vi "Collector Lift.vi"(0 "Collector Lift Man. Value":dbl, 1 "Collector Lift Man.  Request?":bool, 2 "Collector Lift Postion":dbl, 3 "See Portcullis?":bool, 4 "See CDF?":bool, 5 "AutoLift Portcullis?":bool, 6 "Collector Lift States":T1, 7 "AutoAdjust CDF?":bool, 9 "Keep at Target?":bool) -> (20 "Collector Lift Output":dbl, 21 "Collector Lift State Out":T1)   [LabVIEW 2015]
uses:
  Typedefs/CollectorLiftStates.ctl
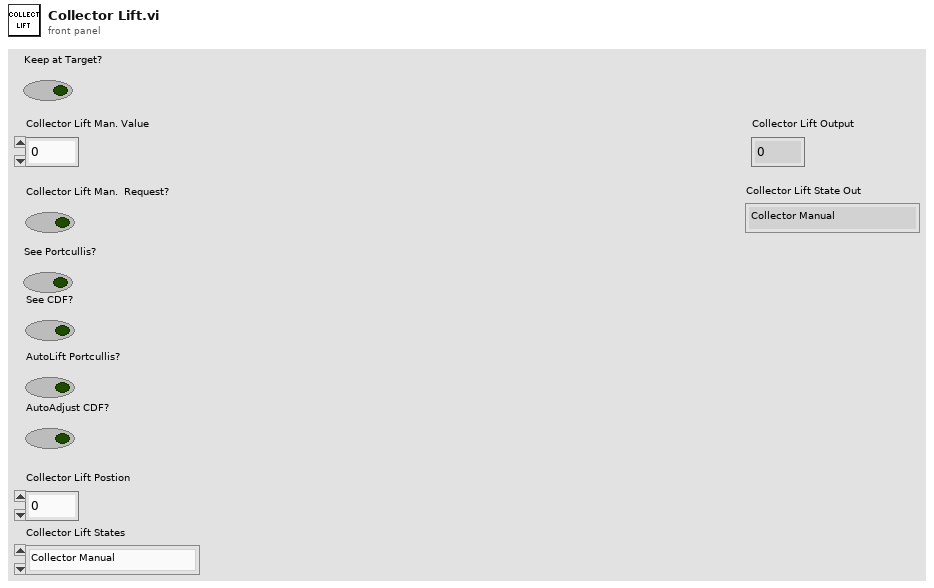
[diagram p1: front panel]
types:
  T1 = typedef "CollectorLiftStates.ctl" = enum16{"Collector Manual", "Stow", "Collect Position", "Spit Position", "Portcullis Set Up", "Portcullis Lift Up", "CDF Set Up", "Push CDF Down"}
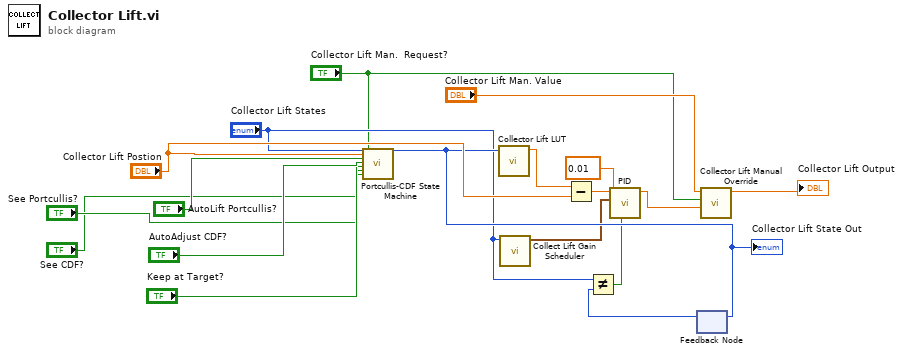
[diagram p0: block diagram]
diagram:
  n1 = call "Portcullis-CDF State Machine.vi"("Collector Lift State"="Collector Lift States", "Collect Lift Position"="Collector Lift Postion", "AutoLift Portcullis?"="AutoLift Portcullis?", "AutoAdjust CDF?"="AutoAdjust CDF?", "Keep at target?"="Keep at Target?", "See Portcullis?"="See Portcullis?", "See CDF?"="See CDF?", "Collector Lift Man.  Request?"="Collector Lift Man.  Request?") -> ("Collector Lift State Out"=w6:T1)  [unwired: 19 in]
  "Collector Lift State Out" <- w6
  n2 = call "Collector Lift LUT.vi"("Collector Lift State"=w6) -> ("Collector Lift Setpoint"=w12:dbl)  [unwired: 10 in]
  n3 = call "Collect Lift Gain Scheduler.vi"("Collector Lift States"="Collector Lift States") -> ("Collect Lift Gains Out"=w2:cluster{"kP":dbl, "kI":dbl, "kD":dbl})  [unwired: 10 in]
  n4 = Subtract(x=w12, y="Collector Lift Postion") -> (x-y=w13:dbl)
  n5 = feedback-in #1(w6) -> ()
  n6 = feedback #1() -> (w5:T1)  [unwired: 1 in]
  n7 = Not Equal?(x="Collector Lift States", y=w5) -> (x != y?=w4:bool)
  n8 = call "PID.vi"("Reset I?"=w4, "Loop Period"=0.01, "Gains"=w2, "Error"=w13) -> ("Output"=w10:dbl)  [unwired: 5 in, 2 out]
  n9 = call "Collector Lift Manual Override.vi"("Output"=w10, "Collector Lift Man.  Request?"="Collector Lift Man.  Request?", "Collector Lift Man. Value"="Collector Lift Man. Value") -> ("Collector Lift Output"=→"Collector Lift Output":dbl)  [unwired: 8 in]
